vi "MEMR-Analyze All.vi"(0 "Files":path[](array[path])=[path "D:/Data/MEMR/Ken/SFMH41-MEMR-1.txt", path "D:/Data/MEMR/Ken/SFMH41-MEMR-2.txt", path "D:/Data/MEMR/Ken/SFMH41-MEMR-3.txt"], 2 "Force reanalyze":bool, 7 "Threshold":T1={"Measure"=enum."at max mag", "T(ms) re peak"=0.0, "Fmin (Hz)"=500.0, "Fmax (Hz)"=5000.0, "Window"=enum."None", "Resol (Hz)"=0.0, "Wpeak (Hz)"=0.0, "Criterion"=0.0, "Compute"=enum."Mean", "Scale"=enum."Linear"}, 11 "Error In":errorcluster) -> (4 "processed":T2, 8 "Threshold (out)":T1, 10 "update threshold":bool, 15 "error out":errorcluster)   [LabVIEW 2020]
uses:
  MEMR-Offline Analysis Parameters.ctl
  MEMR-Processed Data.ctl
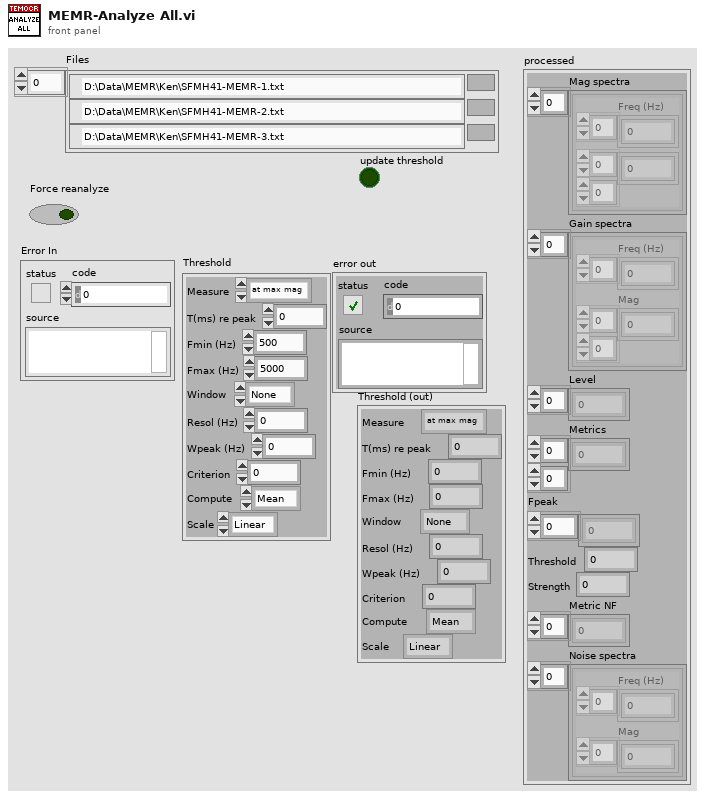
[diagram p1: front panel]
types:
  T1 = typedef "MEMR-Offline Analysis Parameters.ctl" = cluster{"Measure":enum16{"at max mag", "at max gain", "over window", "optimize", "Keefe"}, "T(ms) re peak":dbl, "Fmin (Hz)":dbl, "Fmax (Hz)":dbl, "Window":enum16{"None", "Hanning", "Hamming"}, "Resol (Hz)":dbl, "Wpeak (Hz)":dbl, "Criterion":dbl, "Compute":enum16{"Mean", "Sum"}, "Scale":enum16{"Linear", "Log"}}
  T2 = typedef "MEMR-Processed Data.ctl" = cluster{"Mag spectra":cluster{"Freq (Hz)":dbl[], dbl[][]}[], "Gain spectra":cluster{"Freq (Hz)":dbl[], "Mag":dbl[][]}[], "Level":dbl[], "Metrics":dbl[][], "Fpeak":dbl[], "Threshold":dbl, "Strength":dbl, "Metric NF":dbl[], "Noise spectra":cluster{"Freq (Hz)":dbl[], "Mag":dbl[]}[]}
  T3 = enum16{"at max mag", "at max gain", "over window", "optimize", "Keefe"}
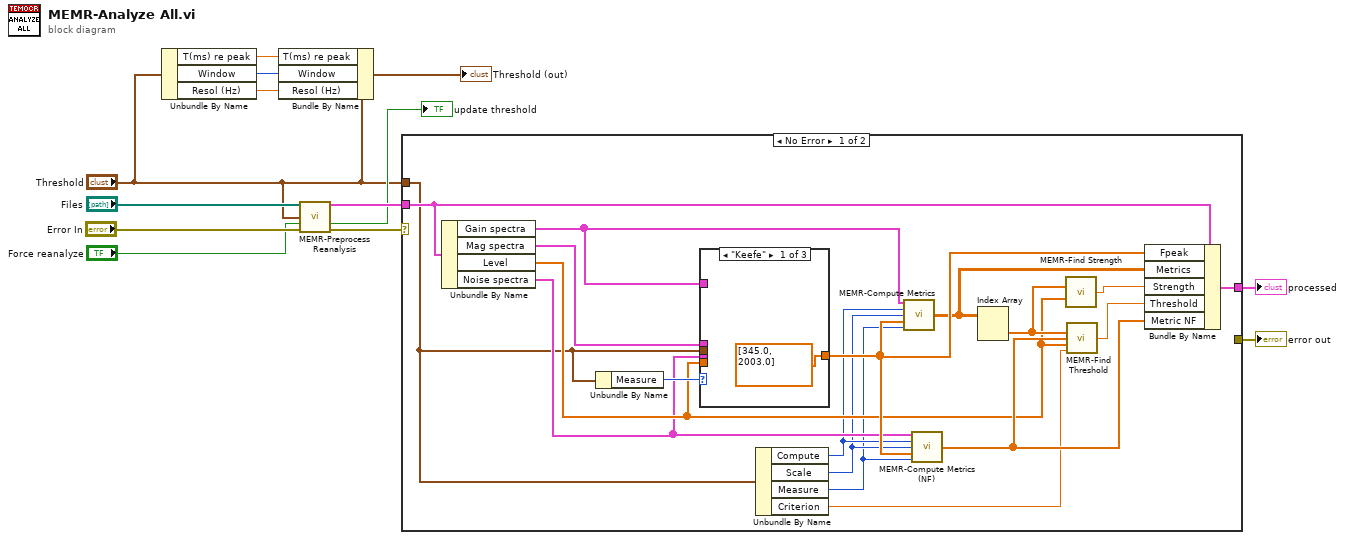
[diagram p0: block diagram]
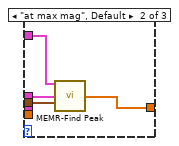
[diagram p2: hidden frame]
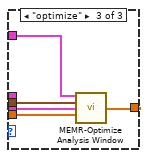
[diagram p3: hidden frame]
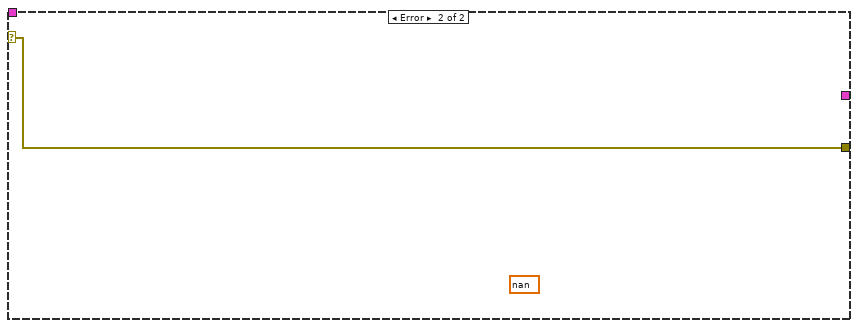
[diagram p4: hidden frame]
diagram:
  n1 = Unbundle By Name("Threshold") -> ("T(ms) re peak"=w3:dbl, "Window"=w2:enum16{"None", "Hanning", "Hamming"}, "Resol (Hz)"=w1:dbl)
  n2 = Bundle By Name(cluster="Threshold", "T(ms) re peak"=w3, "Window"=w2, "Resol (Hz)"=w1) -> (→"Threshold (out)":T1)
  n3 = call "MEMR-Preprocess Reanalysis.vi"("Files"="Files", "Threshold"="Threshold", "Force reanalyze"="Force reanalyze", "Error In"="Error In") -> ("preprocessed"=w10:T2, "update threshold"=→"update threshold":bool, "error out"=w9:errorcluster)  [unwired: 8 in, 1 out]
  n4 = case shown="No Error" w9 {
    selector: w9 -> [_ w42]
    tunnel: "Threshold" -> [w18 _]
    tunnel: [_ w42] -> w13
    tunnel: [w30 _] -> w12
    tunnel: w10 -> [w22 _]
    frame No Error {
      n5 = Unbundle By Name(w22) -> ("Gain spectra"=w23:cluster{"Freq (Hz)":dbl[], "Mag":dbl[][]}[], "Mag spectra"=w20:cluster{"Freq (Hz)":dbl[], dbl[][]}[], "Level"=w21:dbl[], "Noise spectra"=w19:cluster{"Freq (Hz)":dbl[], "Mag":dbl[]}[])
      n6 = Unbundle By Name(w18) -> ("Measure"=w27:T3)
      n7 = case shown="\"Keefe\"" w27 {
        tunnel: w23 -> [_ w36 w41]
        tunnel: w20 -> [_ w35 _]
        tunnel: w19 -> [_ _ w40]
        tunnel: w18 -> [_ w34 w39]
        tunnel: [dbl[] [345.0, 2003.0] ("Fpeak") w33 w38] -> w26
        tunnel: w21 -> [_ _ w37]
        frame "Keefe" {
        }
        frame "at max mag", Default {
          n8 = call "MEMR-Find Peak.vi"("Gain spectra"=w36, "Mag spectra"=w35, "Threshold"=w34) -> ("Fpeak"=w33:dbl[])  [unwired: 12 in]
        }
        frame "optimize" {
          n9 = call "MEMR-Optimize Analysis Window.vi"("Gain spectra"=w41, "Threshold"=w39, "Noise spectra"=w40, "Level"=w37) -> ("Fpeak"=w38:dbl[])  [unwired: 11 in]
        }
      }
      n10 = Unbundle By Name(w18) -> ("Compute"=w16:enum16{"Mean", "Sum"}, "Scale"=w15:enum16{"Linear", "Log"}, "Measure"=w14:T3, "Criterion"=w17:dbl)
      n11 = call "MEMR-Compute Metrics.vi"("Gain spectra in"=w23, "Compute"=w16, "Scale"=w15, "Fpeak"=w26, "Measure"=w14) -> ("Metrics"=w24:dbl[][])  [unwired: 9 in, 1 out]
      n12 = call "MEMR-Compute Metrics (NF).vi"("Gain spectra in"=w19, "Compute"=w16, "Scale"=w15, "Fpeak"=w26, "Measure"=w14) -> ("Metrics"=w25:dbl[])  [unwired: 9 in, 1 out]
      n13 = Index Array(array=w24) -> (element=w28:dbl[])  [unwired: 2 in]
      n14 = call "MEMR-Find Strength.vi"("Metrics"=w28, "Level"=w21) -> ("Strength"=w29:dbl)  [unwired: 13 in]
      n15 = call "MEMR-Find Threshold.vi"("Metrics"=w28, "Noise"=w25, "Level"=w21, "Criterion"=w17) -> ("Threshold"=w31:dbl)  [unwired: 11 in]
      n16 = Bundle By Name(cluster=w22, "Fpeak"=w26, "Metrics"=w24, "Strength"=w29, "Threshold"=w31, "Metric NF"=w25) -> (w30:T2)
    }
    frame Error {
      (unwired) nan ("Threshold")
    }
  }
  "error out" <- w13
  "processed" <- w12
